vi "BumpSetpoint.vi"(8 "Bump Down Trigger":bool, 9 "Bump Up Trigger":bool, 10 "Bump Increment":dbl, 11 "Original Setpoint":dbl) -> (2 "Bumped Setpoint":dbl)   [LabVIEW 2019]
doc: "Bumps a setpoint up or down by a specified interval"
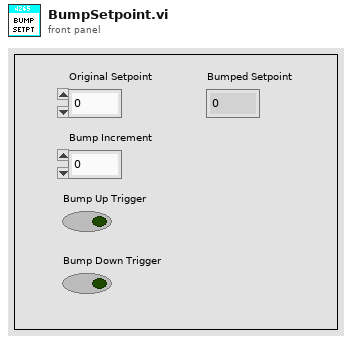
[diagram p1: front panel]
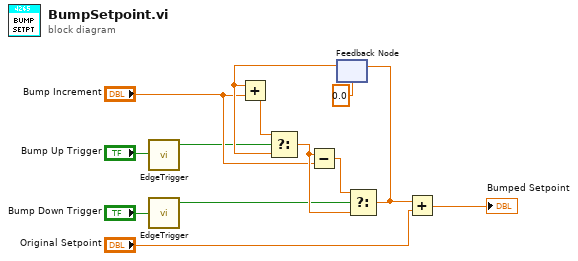
[diagram p0: block diagram]
diagram:
  n1 = call "EdgeTrigger.vi"("Input Signal"="Bump Up Trigger") -> ("Rising Edge Trigger"=w3:bool)  [unwired: 2 out]
  n2 = call "EdgeTrigger.vi"("Input Signal"="Bump Down Trigger") -> ("Rising Edge Trigger"=w1:bool)  [unwired: 2 out]
  n3 = feedback #1(0.0) -> (w11:dbl)
  n4 = Add(x=w11, y="Bump Increment") -> (x+y=w8:dbl)
  n5 = Select(t=w8, s=w3, f=w11) -> (s? t:f=w12:dbl)
  n6 = Subtract(x=w12, y="Bump Increment") -> (x-y=w13:dbl)
  n7 = Select(t=w13, s=w1, f=w12) -> (s? t:f=w7:dbl)
  n8 = feedback-in #1(w7) -> ()
  n9 = Add(x=w7, y="Original Setpoint") -> (x+y=→"Bumped Setpoint":dbl)
